vi "LibreVNA Test 02.vi"() -> ()   [LabVIEW 2023]
uses:
  LibreVNA/Types/Trace Enum.ctl
  LibreVNA/LibreVNA.lvclass
  controls/SData.ctl
panel:
  out "Time Stamp":timestamp format="%<%x %.3X>T"
  out "Exit":bool
  out "size(s)":i32
  in  "command delay (ms)":u32=1000
  out "Numeric":i32
  out "Is Running":bool
  out "XY Graph":cluster{"Data Out":dbl[], "Data Out":dbl[]}(graph)
  in  "Trace Name":T1
  in  "Stop":bool
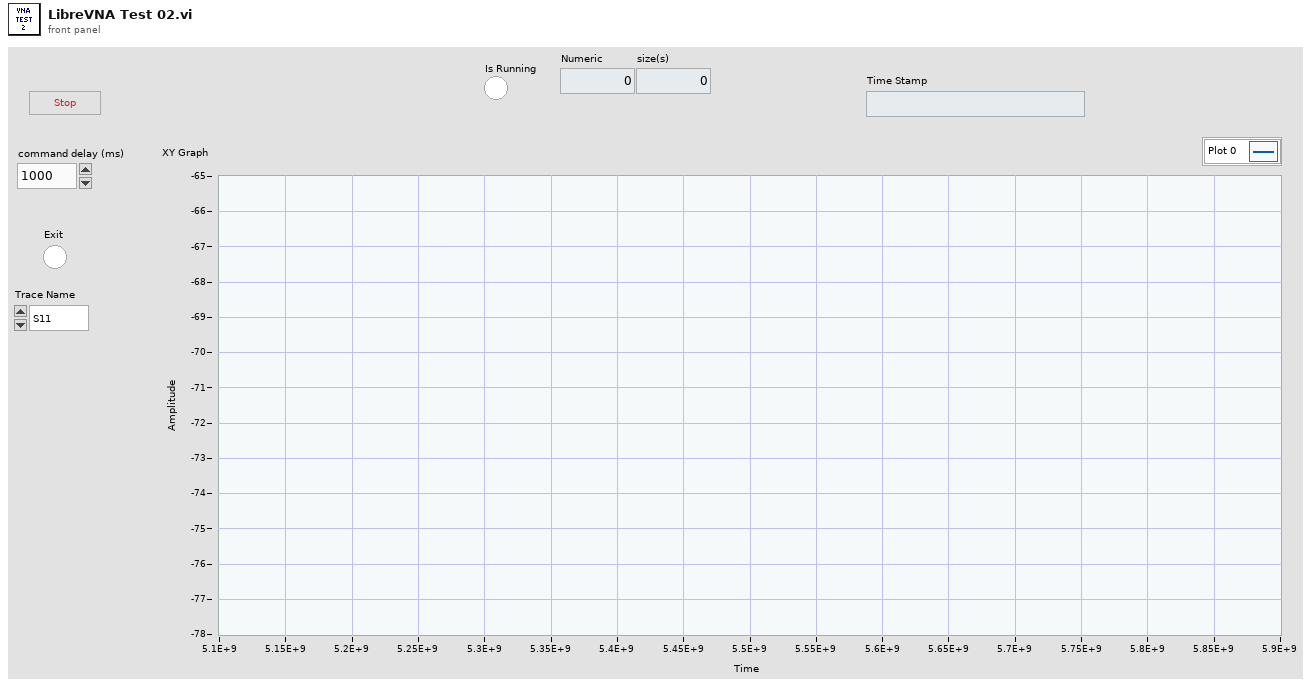
[diagram p1: front panel]
types:
  T1 = typedef "LibreVNA.lvclass/Trace Enum.ctl" = enum16{"S11", "S12", "S21", "S22"}
  T2 = typedef "SData.ctl" = cluster{"Time Stamp":timestamp, "Array":dbl[][]}
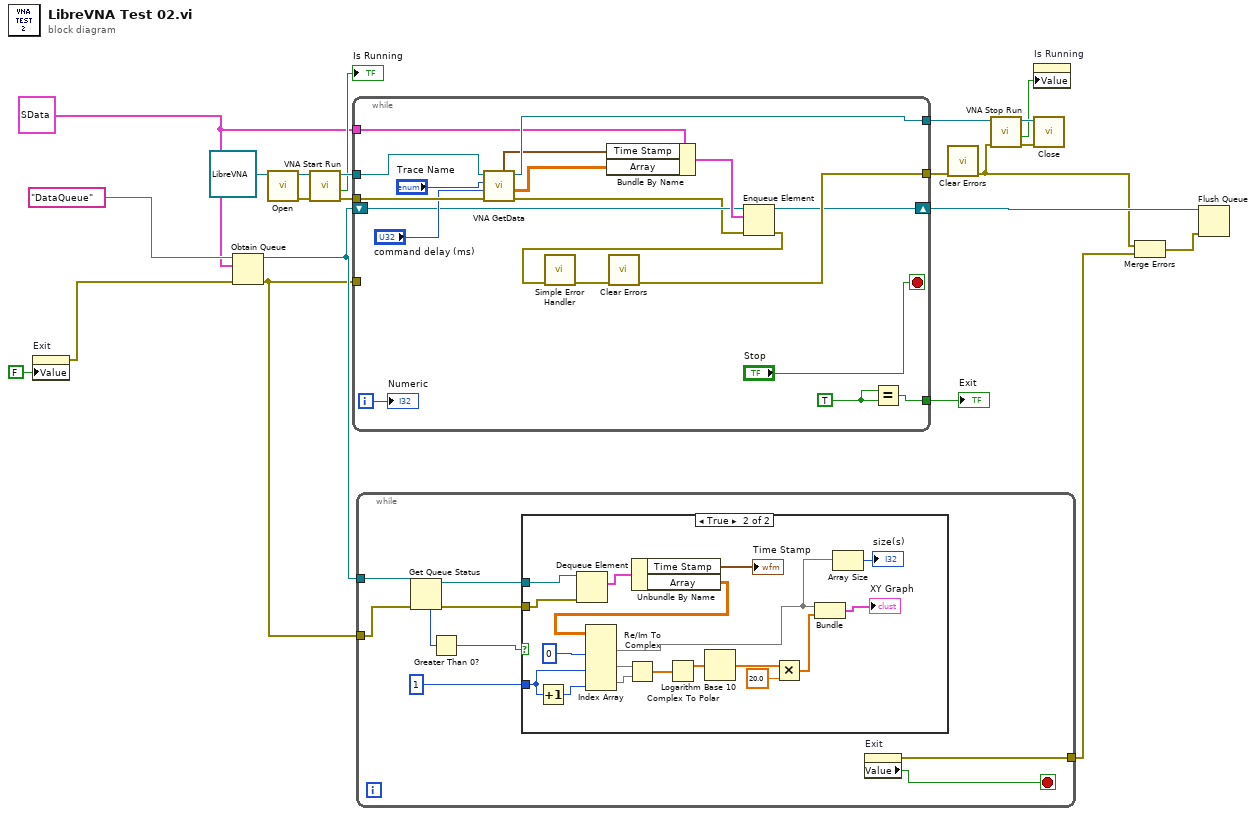
[diagram p0: block diagram]
diagram:
  w10 = T2 {"Time Stamp"=timestamp(0 s since 1904-01-01), "Array"=[]} ("S-Data")
  n1 = property on="Exit" class="Bool (strict)"("Value"=FALSE ("Exit")) -> (error out=w8:errorcluster)  [unwired: 2 in, 1 out]
  n2 = Obtain Queue(name (unnamed)="DataQueue", element data type=w10, error in (no error)=w8) -> (queue out=w9:refnum<queue>, error out=w7:errorcluster)  [unwired: 2 in, 1 out]
  n3 = call-dynamic "Open.vi"("LibreVNA in"=refnum<class "LibreVNA.lvclass"> refnum ("LibreVNA.lvclass")) -> ("error out"=w18:errorcluster, "LibreVNA out"=w21:refnum<class "LibreVNA.lvclass">)  [unwired: 9 in]
  n4 = call-dynamic "VNA Start Run.vi"("error in (no error)"=w18, "LibreVNA in"=w21) -> ("error out"=w17:errorcluster, "Is Running"=→"Is Running":bool, "LibreVNA out"=w19:refnum<class "LibreVNA.lvclass">)  [unwired: 7 in]
  n5 = while {
    tunnel: w17 -> [w41]
    tunnel: w19 -> [w40]
    tunnel: [w38] -> w20
    tunnel: [w39] -> w16
    tunnel: w10 -> [w33]
    tunnel: [w25] -> w5
    tunnel: w7 -> [_]
    shift-right: [w23] -> w4
    shift-left: w9 -> [w29]
    i -> [w35]
    stop <- "Stop" stop-if-true
    w24 = TRUE
    n6 = call-dynamic "VNA GetData.vi"("error in (no error)"=w41, "command delay (ms)"="command delay (ms)", "Trace Name"="Trace Name", "LibreVNA in"=w40) -> ("error out"=w27:errorcluster, "Data Out"=w31:dbl[][], "LibreVNA out"=w39:refnum<class "LibreVNA.lvclass">, "TimeStamp"=w32:timestamp)  [unwired: 2 in, 2 out]
    n7 = Bundle By Name(cluster=w33, "Time Stamp"=w32, "Array"=w31) -> (w30:T2)
    n8 = Enqueue Element(queue=w29, element=w30, error in (no error)=w27) -> (queue out=w23:refnum<queue>, error out=w26:errorcluster)  [unwired: 1 in, 1 out]
    n9 = call <vilib>:"Simple Error Handler.vi"("error in (no error)"=w26) -> ("error out"=w28:errorcluster)  [unwired: 4 in, 4 out]
    n10 = call <vilib>:"Clear Errors.vi"("error in (no error)"=w28) -> ("error out"=w38:errorcluster)  [unwired: 5 in, 1 out]
    n11 = Equal?(x=w24, y=w24) -> (x = y?=w25:bool)
    "Numeric" <- w35
  }
  "Exit" <- w5
  n12 = while {
    tunnel: w9 -> [w49]
    tunnel: w7 -> [w48]
    tunnel: [w42] -> w3
    stop <- w50 stop-if-true
    n13 = Get Queue Status(queue=w49, error in (no error)=w48) -> (queue out=w45:refnum<queue>, error out=w44:errorcluster, # elements in queue=w47:i32)  [unwired: 1 in, 5 out]
    n14 = Greater Than 0?(x=w47) -> (x > 0?=w46:bool)
    n15 = case shown="True" w46 {
      tunnel: w45 -> [_ w63]
      tunnel: w44 -> [_ w62]
      tunnel: 1 ("index (col)") -> [_ w52]
      frame False {
      }
      frame True {
        n16 = Increment(x=w52) -> (x+1=w51:i32)
        n17 = Dequeue Element(queue=w63, error in (no error)=w62) -> (element=w61:T2)  [unwired: 1 in, 3 out]
        n18 = Unbundle By Name(w61) -> ("Time Stamp"=→"Time Stamp":timestamp, "Array"=w59:dbl[][])
        n19 = Index Array(array=w59, index (col) #1=0 ("disabled index (col)"), index (col) #2=w52, index (col) #3=w51) -> (element #1=w54:dbl[], element #2=w58:dbl[], element #3=w57:dbl[])  [unwired: 3 in]
        n20 = Re/Im To Complex(1:w57, 2:w58) -> (0:w66:cdb[])
        n21 = Complex To Polar(r * e^(i*theta)=w66) -> (r=w67:dbl[])  [unwired: 1 out]
        n22 = Logarithm Base 10(1:w67) -> (0:w68:dbl[])
        n23 = Multiply(x=w68, y=20.0) -> (x*y=w56:dbl[])
        n24 = Bundle("Array"=w54, w56) -> (→"XY Graph":cluster{"Array":dbl[], dbl[]})  [unwired: 1 in]
        n25 = Array Size(array=w54) -> (size(s)=→"size(s)":i32)
      }
    }
    n26 = property on="Exit" class="Bool (strict)"() -> (error out=w42:errorcluster, "Value"=w50:bool)  [unwired: 2 in, 1 out]
  }
  n27 = call <vilib>:"Clear Errors.vi"("error in (no error)"=w20) -> ("error out"=w2:errorcluster)  [unwired: 5 in, 1 out]
  n28 = call-dynamic "VNA Stop Run.vi"("error in (no error)"=w2, "LibreVNA in"=w16) -> ("error out"=w14:errorcluster, "Is Running"=w12:bool, "LibreVNA out"=w15:refnum<class "LibreVNA.lvclass">)  [unwired: 7 in]
  n29 = property on="Is Running" class="Bool (strict)"("Value"=w12) -> ()  [unwired: 2 in, 2 out]
  n30 = call-dynamic "Close.vi"("error in (no error)"=w14, "LibreVNA in"=w15) -> ()  [unwired: 8 in, 2 out]
  n31 = Merge Errors(w2, w3) -> (w1:errorcluster)
  n32 = Flush Queue(queue=w4, error in (no error)=w1) -> ()  [unwired: 3 out]
